vi "Unpack Nested Value Update.vi"(11 "Nested Value Update Msg":refnum<class "Nested Value Update Msg.lvclass">) -> (0 "Value":variant, 1 "Time":u32, 2 "Datum Name":string)   [LabVIEW 2020, in "MVA Framework.lvlib" / "IViewable.lvlib" / "Nested Value Update Msg.lvclass"]
uses:
  Nested Value Update Msg.lvclass
  Nested Value Update Msg.lvclass/Nested Value Update Msg.ctl
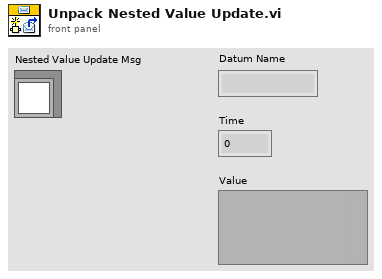
[diagram p1: front panel]
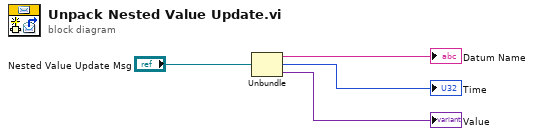
[diagram p0: block diagram]
diagram:
  n1 = Unbundle("Nested Value Update Msg") -> (→"Datum Name":string, →"Time":u32, →"Value":variant)
